vi "SynapseAPI-Set Parameter Value (DBL).vi"(0 "URL":string="http://localhost:24414", 5 "Gizmo":string, 7 "Parameter":string, 9 "Value":dbl, 11 "error in (no error)":errorcluster) -> (15 "error out":errorcluster)   [LabVIEW 2015]
uses:
  <vilib>/httpClient/PUTBuffer.vi
  <vilib>/httpClient/LabVIEWHTTPClient.lvlib
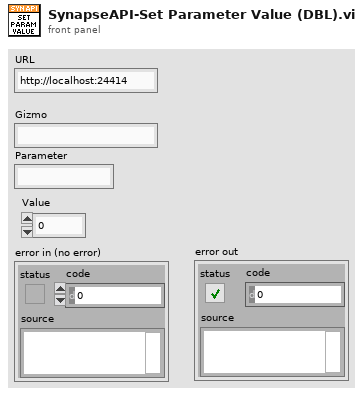
[diagram p1: front panel]
types:
  T1 = typedef "LabVIEWHTTPClient.lvlib/ClientHandle.ctl" = refnum<k1>
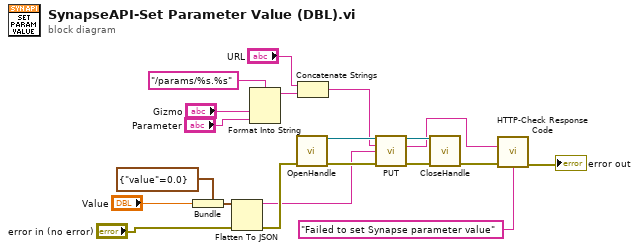
[diagram p0: block diagram]
diagram:
  n1 = Bundle(cluster=cluster{"value":dbl} {"value"=0.0} ("Cluster"), "value"="Value") -> (w8:cluster{"value":dbl})
  n2 = Flatten To JSON(anything=w8, error in (no error)="error in (no error)") -> (JSON string=w5:string, 11:w6:errorcluster)  [unwired: 1 in]
  n3 = Format Into String(format string="/params/%s.%s", "Gizmo", "Parameter") -> (resulting string=w14:string)  [unwired: 2 in, 1 out]
  n4 = call <vilib>:"OpenHandle.vi"("error in (no error)"=w6) -> ("client handle out"=w18:T1, "error out"=w17:errorcluster)  [unwired: 13 in]
  n5 = Concatenate Strings("URL", w14) -> (w16:string)
  n6 = call-poly <vilib>:"PUT.vi"("client handle"=w18, "url"=w16, "buffer"=w5, "error in (no error)"=w17) -> ("client handle out"=w19:T1, "headers"=w3:string, "error out"=w20:errorcluster)  [unwired: 8 in, 1 out]
  n7 = call <vilib>:"CloseHandle.vi"("client handle"=w19, "error in (no error)"=w20) -> ("error out"=w4:errorcluster)  [unwired: 13 in]
  n8 = call "HTTP-Check Response Code.vi"("headers"=w3, "error in"=w4, "message"="Failed to set Synapse parameter value" ("source")) -> ("error out"=→"error out":errorcluster)  [unwired: 12 in]
